vi "Tower Light Status.vi"(2 "Enum":enum16{"Idle", "Red Buzzer", "Yello", "Green"}(ring)) -> ()   [LabVIEW 2015]
uses:
  Galobal variable_TI.vi
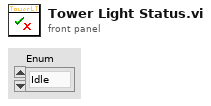
[diagram p1: front panel]
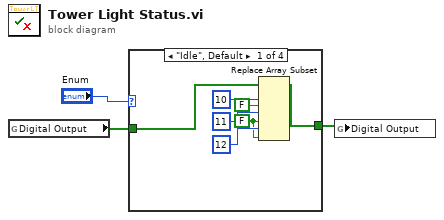
[diagram p0: block diagram]
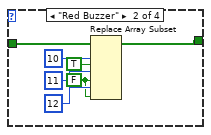
[diagram p2: hidden frame]
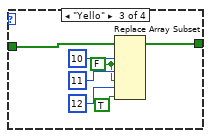
[diagram p3: hidden frame]
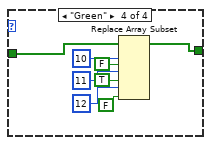
[diagram p4: hidden frame]
diagram:
  n1 = global read "Galobal variable_TI.vi" "Digital Output"() -> (w3:bool[])
  n2 = case shown="\"Idle\", Default" "Enum" {
    tunnel: w3 -> [w5 w17 w20 w27]
    tunnel: [w4 w11 w18 w25] -> w1
    frame "Idle", Default {
      w6 = FALSE ("new element/subarray")
      n3 = Replace Array Subset(array=w5, new element #1=FALSE ("new element/subarray"), index #1=10 ("index"), new element #2=w6, index #2=11 ("index"), new element #3=w6, index #3=12 ("index")) -> (w4:bool[])
    }
    frame "Red Buzzer" {
      w12 = FALSE ("new element/subarray")
      n4 = Replace Array Subset(array=w17, new element #1=TRUE ("new element/subarray"), index #1=10 ("index"), new element #2=w12, index #2=11 ("index"), new element #3=w12, index #3=12 ("index")) -> (w11:bool[])
    }
    frame "Yello" {
      w19 = FALSE ("new element/subarray")
      n5 = Replace Array Subset(array=w20, new element #1=w19, index #1=10 ("index"), new element #2=w19, index #2=11 ("index"), new element #3=TRUE ("new element/subarray"), index #3=12 ("index")) -> (w18:bool[])
    }
    frame "Green" {
      n6 = Replace Array Subset(array=w27, new element #1=FALSE ("new element/subarray"), index #1=10 ("index"), new element #2=TRUE ("new element/subarray"), index #2=11 ("index"), new element #3=FALSE ("new element/subarray"), index #3=12 ("index")) -> (w25:bool[])
    }
  }
  n7 = global write "Galobal variable_TI.vi" "Digital Output"(w1) -> ()
